vi "arm driver control.vi"(1 "Joystick Y":dbl) -> (0 "Setpoint":dbl)   [LabVIEW 2013]
uses:
  typedefs/fg_typedef.ctl
  typedefs/DevRef Type.ctl
panel:
  # "Control the arm with PID setpoints instead of direct motor control"
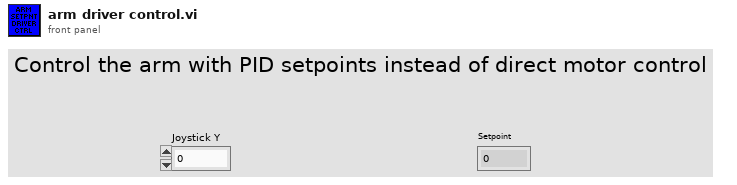
[diagram p1: front panel]
types:
  T1 = typedef "DevRef Type.ctl" = enum16{"Shooter Solenoid", "Latch Solenoid", "Right Up Sensor", "Right Down Sensor", "Hold Sensor", "Arm Encoder"}
  T2 = typedef "fg_typedef.ctl" = enum16{"Get", "Set"}
  T3 = typedef "WPI_EncoderDevRef.ctl" = cluster{"DevStatus":errorcluster, "EncoderIndex":T4, "CounterIndex":T5, "DistancePerCount":dbl, "Decoding Type":T6}
  T4 = typedef "FPGA_EncoderIdx.ctl" = enum8{"Enc 0", "Enc 1", "Enc 2", "Enc 3", "Invalid"}
  T5 = typedef "FPGA_CounterCtrSystemIndex.ctl" = enum8{"Ctr 0", "Ctr 1", "Ctr 2", "Ctr 3", "Ctr 4", "Ctr 5", "Ctr 6", "Ctr 7", "Invalid"}
  T6 = typedef "WPI_EncoderType.ctl" = enum16{"1x", "2x", "4x"}
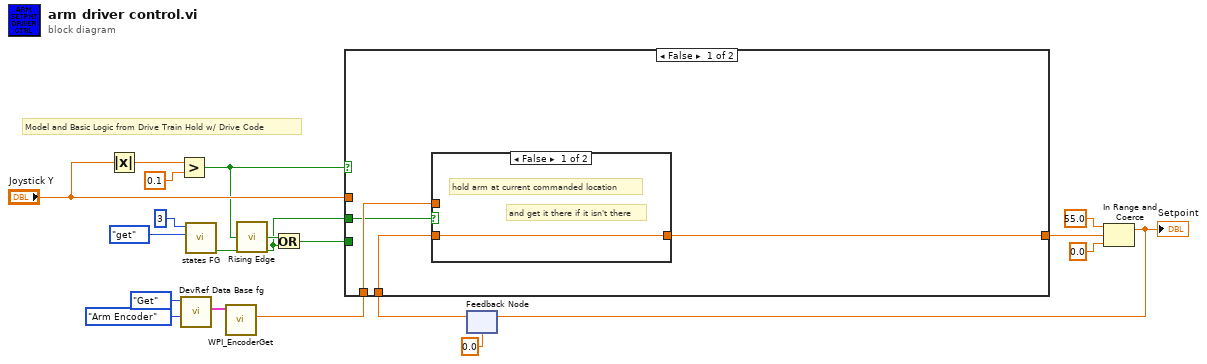
[diagram p0: block diagram]
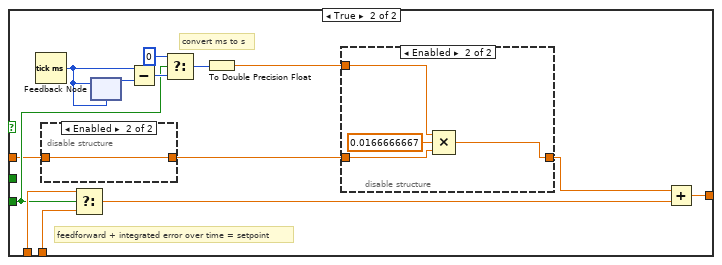
[diagram p3: hidden frame]
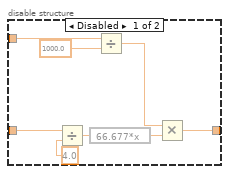
[diagram p4: hidden frame]
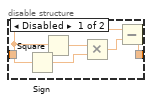
[diagram p5: hidden frame]
diagram:
  # "Model and Basic Logic from Drive Train Hold w/ Drive Code"
  n1 = Absolute Value(x="Joystick Y") -> (abs(x)=w15:dbl)
  n2 = Greater?(x=w15, y=0.1) -> (0:w8:bool)
  n3 = call "DevRef Data Base fg.vi"("DevRef to Get"=DevRef_Type."Arm Encoder", "Menu"=fg_typedef."Get") -> ("Selected Encoder"=w10:T3)  [unwired: 1 in, 8 out]
  n4 = call "states FG.vi"("menu (get)"=enum16{"set", "get"}."get", "Loop ID"=3) -> ("first call?"=w3:bool)  [unwired: 6 in, 3 out]
  n5 = call <vilib>:"WPI_EncoderGet.vi"("EncoderDevRef"=w10) -> ("Distance"=w7:dbl)  [unwired: 5 in, 5 out]
  n6 = call "Rising Edge.vi"("Input"=w8) -> ("Rising Edge"=w11:bool)
  n7 = Or(x=w11, y=w3) -> (x .or. y?=w5:bool)
  n8 = feedback #1(0.0 ("upper limit")) -> (w6:dbl)
  n9 = case shown="False" w8 {
    tunnel: "Joystick Y" -> [_ w32]
    tunnel: w6 -> [w23 w37]
    tunnel: w5 -> [_ w33]
    tunnel: w7 -> [w22 w36]
    tunnel: [w21 w30] -> w4
    tunnel: w3 -> [w20 _]
    frame False {
      n10 = case shown="False" w20 {
        tunnel: w23 -> [w24 _]
        tunnel: w22 -> [_ w25]
        tunnel: [w24 w25] -> w21
        frame False {
          # "and get it there if it isn't there"
          # "hold arm at current commanded location"
        }
        frame True {
          # "hold arm at encoder location"
        }
      }
    }
    frame True {
      # "feedforward + integrated error over time = setpoint"
      # "convert ms to s"
      n11 = Tick Count (ms)() -> (millisecond timer value=w27:u32)
      n12 = disable-structure shown="Enabled" {
        disable-tunnel: w32 -> [w56 w57]
        disable-tunnel: [w55 w57] -> w29
        frame Disabled {
          n13 = Sign(1:w56) -> (0:w53:dbl)
          n14 = Square(x=w56) -> (x^2=w54:dbl)
          n15 = Multiply(x=w54, y=w53) -> (x*y=w52:dbl)
          n16 = Subtract(x=w56, y=w52) -> (x-y=w55:dbl)
        }
        frame Enabled {
        }
      }
      n17 = Select(t=w36, s=w33, f=w37) -> (s? t:f=w31:dbl)
      n18 = feedback #2(w27) -> (w28:u32)
      n19 = feedback-in #2(w27) -> ()
      n20 = Subtract(x=w27, y=w28) -> (x-y=w38:u32)
      n21 = Select(t=u32 0, s=w33, f=w38) -> (s? t:f=w34:u32)
      n22 = To Double Precision Float(number=w34) -> (double precision float=w35:dbl)
      n23 = disable-structure shown="Enabled" {
        disable-tunnel: w35 -> [w47 w51]
        disable-tunnel: w29 -> [w43 w50]
        disable-tunnel: [w40 w48] -> w26
        frame Disabled {
          n24 = Divide(x=w43, y=4.0) -> (x/y=w42:dbl)
          n25 = expression code="66.677*x"(w42) -> (w41:dbl)
          n26 = Divide(x=w47, y=1000.0) -> (x/y=w45:dbl)
          n27 = Multiply(x=w45, y=w41) -> (x*y=w40:dbl)
        }
        frame Enabled {
          n28 = Compound Arithmetic op=MULTIPLY(w51, 0.0166666667 ("value"), w50) -> (w48:dbl)
        }
      }
      n29 = Add(x=w26, y=w31) -> (x+y=w30:dbl)
    }
  }
  n30 = In Range and Coerce(upper limit=55.0, x=w4, lower limit=0.0) -> (coerced(x)=w17:dbl)  [unwired: 1 out]
  "Setpoint" <- w17
  n31 = feedback-in #1(w17) -> ()
